vi "generate complex plane region.vi"(7 "number of grid points":i32, 8 "center im":dbl, 9 "center re":dbl, 10 "delta im":dbl, 11 "delta re":dbl) -> (3 "complex region":cdb[][](array[numeric]))   [LabVIEW 2010]
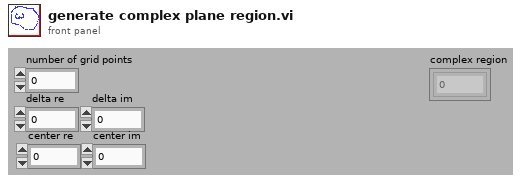
[diagram p1: front panel]
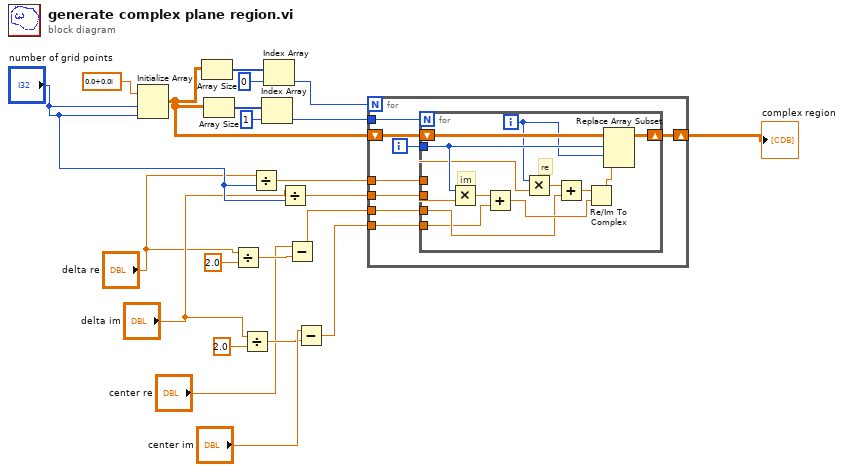
[diagram p0: block diagram]
diagram:
  n1 = Initialize Array(cdb 0.0+0.0i ("element"), "number of grid points", "number of grid points") -> (w15:cdb[][])
  n2 = Array Size(array=w15) -> (size(s)=w21:i32[])
  n3 = Array Size(array=w15) -> (size(s)=w18:i32[])
  n4 = Divide(x="delta re", y=2.0) -> (x/y=w4:dbl)
  n5 = Divide(x="delta im", y=2.0) -> (x/y=w7:dbl)
  n6 = Divide(x="delta re", y="number of grid points") -> (x/y=w14:dbl)
  n7 = Index Array(array=w18, index=1) -> (element=w16:i32)
  n8 = Index Array(array=w21, index=0) -> (element=w19:i32)
  n9 = Divide(x="delta im", y="number of grid points") -> (x/y=w13:dbl)
  n10 = Subtract(x="center re", y=w4) -> (x-y=w3:dbl)
  n11 = Subtract(x="center im", y=w7) -> (x-y=w6:dbl)
  n12 = for {
    N: w19 -> [_]
    tunnel: w16 -> [w30]
    shift-right: [w27] -> w11
    shift-left: w15 -> [w29]
    tunnel: w14 -> [w26]
    tunnel: w3 -> [w25]
    tunnel: w13 -> [w24]
    tunnel: w6 -> [w23]
    i -> [w28]
    n13 = for {
      N: w30 -> [_]
      tunnel: w28 -> [w42]
      shift-right: [w40] -> w27
      shift-left: w29 -> [w43]
      tunnel: w26 -> [w34]
      tunnel: w25 -> [w33]
      tunnel: w24 -> [w32]
      tunnel: w23 -> [w31]
      i -> [w41]
      # "re"
      # "im"
      n14 = Multiply(x=w42, y=w32) -> (x*y=w36:dbl)
      n15 = Add(x=w36, y=w31) -> (x+y=w35:dbl)
      n16 = Multiply(x=w41, y=w34) -> (x*y=w38:dbl)
      n17 = Add(x=w38, y=w33) -> (x+y=w37:dbl)
      n18 = Re/Im To Complex(1:w35, 2:w37) -> (0:w39:cdb)
      n19 = Replace Array Subset(array=w43, new element=w39, index (row)=w42, index (col)=w41) -> (w40:cdb[][])
    }
  }
  "complex region" <- w11
